vi "Global INIT.vi"() -> ()   [LabVIEW 2023]
uses:
  ctrl defs/ctrl arm motor.ctl
  ctrl defs/ctrl swerve motor.ctl
  ctrl defs/ctrl MOTOR SELECT.ctl
  <vilib>/Rock Robotics/WPI/ThirdParty/REV Robotics/REVLib/Typedef/Spark MAX Idle Mode.ctl
  ctrl defs/ctrl Spark MAX current limiting.ctl
  ctrl defs/ctrl motor PIDF coefficients.ctl
  <vilib>/Rock Robotics/WPI/ThirdParty/REV Robotics/REVLib/Typedef/Spark MAX Smart Motion Parameters.ctl
  ctrl defs/ctrl limit polarity.ctl
  <vilib>/Rock Robotics/WPI/ThirdParty/REV Robotics/REVLib/Typedef/Spark MAX Limit Switch Polarity.ctl
  ctrl defs/ctrl Talon FX config.ctl
  <vilib>/Rock Robotics/WPI/ThirdParty/Phoenix-LabVIEW/Motor Controller/Controls/CTRE_Phoenix_MotorControl_TalonFXInvertType.ctl
  <vilib>/Rock Robotics/WPI/ThirdParty/Phoenix-LabVIEW/Motor Controller/Controls/CTRE_Phoenix_MotorControl_NeutralMode.ctl
  ctrl defs/ctrl CANcoder.ctl
  ctrl defs/ctrl robot CG.ctl
  ctrl defs/ctrl XY coord.ctl
  ctrl defs/ctrl robot swerve dims.ctl
  ctrl defs/ctrl compressor begin.ctl
  ctrl defs/ctrl compressor config.ctl
  <vilib>/Rock Robotics/WPI/Compressor/WPI_CompressorFeedbackMode.ctl
  ctrl defs/ctrl solenoid.ctl
  <vilib>/Rock Robotics/WPI/Solenoid/WPI_SolenoidChannel.ctl
  <vilib>/Rock Robotics/WPI/Solenoid/WPI_SolenoidValue.ctl
  ctrl defs/ctrl DIO.ctl
  <vilib>/Rock Robotics/SystemInterfaces/DIO/FPGA_DIOChannel.ctl
  ctrl defs/ctrl LED init.ctl
  <vilib>/Rock Robotics/SystemInterfaces/DIO/FPGA_DIOPWMChannel.ctl
  ctrl defs/ctrl number of LEDs.ctl
  ctrl defs/ctrl LED PATTERNS.ctl
  ctrl defs/ctrl DEFINE GEAR.ctl
  ctrl defs/ctrl intake speeds.ctl
  ctrl defs/ctrl shooter speeds.ctl
  ctrl defs/ctrl LIMELIGHT initialize.ctl
  ctrl defs/ctrl ctre pigeon2 config.ctl
  <vilib>/Rock Robotics/WPI/ThirdParty/Phoenix-LabVIEW/Pigeon2/controls/CTRE_Phoenix_Pigeon2_Configurables.ctl
panel:
  in  "Tab Control":T1(tab)
  in  "swerve DRIVE motors":T2[](array[typedef])=[{"refnum name"="front right", "CAN ID"=3, "Installed?"=TRUE, "description"="DRIVE - front right ", "MOTOR SELECT"=6000, "CAN Bus"="SWERVE", "Invert Type"=enum."Counter-Clockwise", "Neutral Mode"=enum."Override to Coast", "gear ratio"=6.75, "MOTOR PIDF coefficients"={"PIDF"={"P Gain"=0.001, "I Gain"=0.0, "D Gain"=0.0, "F Gain"=0.0012, "I Zone"=0.0, "Min Output"=-1.0, "Max Output"=1.0}, "Smart Motion"={"Max Velocity"=1900.0, "Max Acceleration"=750.0, "Minimum Velocity Output"=0.1, "Allowed Closed Loop Error"=0.02}}, "Throttle"={"Ramp Open (s)"=0.0, "Ramp Closed (s)"=0.0, "Percent Deadband"=0.0}, "Supply Current Limits"={"Enable?"=FALSE, "Current Limit"=0.0, "Threshold Current"=0.0, "Threshold Time"=0.0}}, {"refnum name"="front left", "CAN ID"=6, "Installed?"=TRUE, "description"="DRIVE - front left", "MOTOR SELECT"=6000, "CAN Bus"="SWERVE", "Invert Type"=enum."Counter-Clockwise", "Neutral Mode"=enum."Override to Coast", "gear ratio"=6.75, "MOTOR PIDF coefficients"={"PIDF"={"P Gain"=0.001, "I Gain"=0.0, "D Gain"=0.0, "F Gain"=0.0012, "I Zone"=0.0, "Min Output"=-1.0, "Max Output"=1.0}, "Smart Motion"={"Max Velocity"=1900.0, "Max Acceleration"=750.0, "Minimum Velocity Output"=0.1, "Allowed Closed Loop Error"=0.02}}, "Throttle"={"Ramp Open (s)"=0.0, "Ramp Closed (s)"=0.0, "Percent Deadband"=0.0}, "Supply Current Limits"={"Enable?"=FALSE, "Current Limit"=0.0, "Threshold Current"=0.0, "Threshold Time"=0.0}}, {"refnum name"="rear left", "CAN ID"=9, "Installed?"=TRUE, "description"="DRIVE - rear left", "MOTOR SELECT"=6000, "CAN Bus"="SWERVE", "Invert Type"=enum."Counter-Clockwise", "Neutral Mode"=enum."Override to Coast", "gear ratio"=6.75, "MOTOR PIDF coefficients"={"PIDF"={"P Gain"=0.001, "I Gain"=0.0, "D Gain"=0.0, "F Gain"=0.0012, "I Zone"=0.0, "Min Output"=-1.0, "Max Output"=1.0}, "Smart Motion"={"Max Velocity"=1900.0, "Max Acceleration"=750.0, "Minimum Velocity Output"=0.1, "Allowed Closed Loop Error"=0.02}}, "Throttle"={"Ramp Open (s)"=0.0, "Ramp Closed (s)"=0.0, "Percent Deadband"=0.0}, "Supply Current Limits"={"Enable?"=FALSE, "Current Limit"=0.0, "Threshold Current"=0.0, "Threshold Time"=0.0}}, {"refnum name"="rear right", "CAN ID"=12, "Installed?"=TRUE, "description"="DRIVE - rear right", "MOTOR SELECT"=6000, "CAN Bus"="SWERVE", "Invert Type"=enum."Counter-Clockwise", "Neutral Mode"=enum."Override to Coast", "gear ratio"=6.75, "MOTOR PIDF coefficients"={"PIDF"={"P Gain"=0.001, "I Gain"=0.0, "D Gain"=0.0, "F Gain"=0.0012, "I Zone"=0.0, "Min Output"=-1.0, "Max Output"=1.0}, "Smart Motion"={"Max Velocity"=1900.0, "Max Acceleration"=750.0, "Minimum Velocity Output"=0.1, "Allowed Closed Loop Error"=0.02}}, "Throttle"={"Ramp Open (s)"=0.0, "Ramp Closed (s)"=0.0, "Percent Deadband"=0.0}, "Supply Current Limits"={"Enable?"=FALSE, "Current Limit"=0.0, "Threshold Current"=0.0, "Threshold Time"=0.0}}] {"gear ratio" format="%_5f"; "MOTOR SELECT" items=["REV NEO"=5676, "REV NEO 550"=11000, "VEX Falcon"=6380, "WC Kraken"=6000]}
  in  "DRIVE\nwheel diam (in)":dbl=4.0 format="%_4f"
  in  "swerve CANcoders":T8[](array[typedef])=[{"description"="ENC - front right", "Installed?"=TRUE, "CAN ID"=2, "CAN Bus"="SWERVE", "refnum name"="FR ENC", "Sensor Direction"=FALSE, "Magnet Offset (Degrees)"=-264.1113, "gear ratio"=1.0}, {"description"="ENC - front left", "Installed?"=TRUE, "CAN ID"=5, "CAN Bus"="SWERVE", "refnum name"="FL ENC", "Sensor Direction"=FALSE, "Magnet Offset (Degrees)"=-277.20703, "gear ratio"=1.0}, {"description"="ENC - rear left", "Installed?"=TRUE, "CAN ID"=8, "CAN Bus"="SWERVE", "refnum name"="RL ENC", "Sensor Direction"=FALSE, "Magnet Offset (Degrees)"=-124.014, "gear ratio"=1.0}, {"description"="ENC - rear right", "Installed?"=TRUE, "CAN ID"=11, "CAN Bus"="SWERVE", "refnum name"="RR ENC", "Sensor Direction"=FALSE, "Magnet Offset (Degrees)"=-162.158, "gear ratio"=1.0}] {"gear ratio" format="%_5f"}
  in  "swerve STEER motors":T9[](array[typedef])=[{"description"="STEER - front right", "MOTOR SELECT"=5676, "Installed?"=TRUE, "CAN ID"=4, "refnum name"="FR STEER", "Invert"=TRUE, "Idle Mode"=enum."Brake", "Current limiting"={"Linearized"=FALSE, "Free Speed (A)"=20.0, "Primay (A)"=40.0, "Limit RPM (0)"=0}, "MOTOR PIDF coefficients"={"PIDF"={"P Gain"=0.005, "I Gain"=0.0, "D Gain"=0.0, "F Gain"=0.0036, "I Zone"=0.0, "Min Output"=-1.0, "Max Output"=1.0}, "Smart Motion"={"Max Velocity"=1500.0, "Max Acceleration"=750.0, "Minimum Velocity Output"=0.1, "Allowed Closed Loop Error"=0.02}}, "gear ratio"=21.42857}, {"description"="STEER - front left", "MOTOR SELECT"=5676, "Installed?"=TRUE, "CAN ID"=7, "refnum name"="FL STEER", "Invert"=TRUE, "Idle Mode"=enum."Brake", "Current limiting"={"Linearized"=FALSE, "Free Speed (A)"=20.0, "Primay (A)"=40.0, "Limit RPM (0)"=0}, "MOTOR PIDF coefficients"={"PIDF"={"P Gain"=0.005, "I Gain"=0.0, "D Gain"=0.0, "F Gain"=0.0036, "I Zone"=0.0, "Min Output"=-1.0, "Max Output"=1.0}, "Smart Motion"={"Max Velocity"=1500.0, "Max Acceleration"=750.0, "Minimum Velocity Output"=0.1, "Allowed Closed Loop Error"=0.02}}, "gear ratio"=21.429}, {"description"="STEER - rear left", "MOTOR SELECT"=5676, "Installed?"=TRUE, "CAN ID"=10, "refnum name"="RL STEER", "Invert"=TRUE, "Idle Mode"=enum."Brake", "Current limiting"={"Linearized"=FALSE, "Free Speed (A)"=20.0, "Primay (A)"=40.0, "Limit RPM (0)"=0}, "MOTOR PIDF coefficients"={"PIDF"={"P Gain"=0.005, "I Gain"=0.0, "D Gain"=0.0, "F Gain"=0.0036, "I Zone"=0.0, "Min Output"=-1.0, "Max Output"=1.0}, "Smart Motion"={"Max Velocity"=1500.0, "Max Acceleration"=750.0, "Minimum Velocity Output"=0.1, "Allowed Closed Loop Error"=0.02}}, "gear ratio"=21.42857}, {"description"="STEER - rear right", "MOTOR SELECT"=5676, "Installed?"=TRUE, "CAN ID"=13, "refnum name"="RR STEER", "Invert"=TRUE, "Idle Mode"=enum."Brake", "Current limiting"={"Linearized"=FALSE, "Free Speed (A)"=20.0, "Primay (A)"=40.0, "Limit RPM (0)"=0}, "MOTOR PIDF coefficients"={"PIDF"={"P Gain"=0.005, "I Gain"=0.0, "D Gain"=0.0, "F Gain"=0.0036, "I Zone"=0.0, "Min Output"=-1.0, "Max Output"=1.0}, "Smart Motion"={"Max Velocity"=1500.0, "Max Acceleration"=750.0, "Minimum Velocity Output"=0.1, "Allowed Closed Loop Error"=0.02}}, "gear ratio"=21.42857}] {"gear ratio" format="%_5f"; "MOTOR SELECT" items=["REV NEO"=5676, "REV NEO 550"=11000, "VEX Falcon"=6380, "WC Kraken"=6000]}
  in  "PIGEON":T12={"Installed?"=TRUE, "Configurables"={"Mount Pose Yaw"=0.0, "Mount Pose Pitch"=0.0, "Mount Pose Roll"=0.0, "Disable Temperature Compensation"=FALSE, "Disable No-Motion Calibration"=FALSE, "Enable Compass"=TRUE}, "CAN ID"=1, "refnum name"="PIGEON2", "CAN bus"="SWERVE"}
  in  "LIMELIGHT":T14={"Installed?"=TRUE, "pose"={"X"=0.0, "Y"=-3.0, "Z"=23.0, "angle to horizon"=-34.5, "tx angle offset"=0.0}}
  in  "LED init":T15={"PWM Channel"=enum."PWM 1", "refnum name"="LED", "#LEDS"=120, "initial output"=0.51, "stack name"="LED/value", "Installed?"=TRUE, "pattern"=0} {"pattern" items=["<<Select a pattern>>", "Rainbow, Rainbow palette", "Rainbow, Party palette", "Rainbow, Ocean palette", "Rainbow, Lava palette", "Rainbow, Forest palette", "Rainbow with glitter", "Confetti", "Shot, Red", "Shot, Blue", "Shot, White", "Sinelon, Rainbow palette", "Sinelon, Party palette", "Sinelon, Ocean palette", "Sinelon, Lava palette", "Sinelon, Forest palette", "BPM, Rainbow palette", "BPM, Party palette", "BPM, Ocean palette", "BPM, Lava palette", "BPM, Forest palette", "Fire, Medium", "Fire, Large", "Twinkles, Rainbow palette", "Twinkles, Party palette", "Twinkles, Ocean palette", "Twinkles, Lava palette", "Twinkles, Forest palette", "Color Waves, Rainbow palette", "Color Waves, Party palette", "Color Waves, Ocean palette", "Color Waves, Lava palette", "Color Waves, Forest palette", "Larson Scanner, Red", "Larson Scanner, Gray", "Light Chase, Red", "Light Chase, Blue", "Light Chase, Gray", "Heartbeat, Red", "Heartbeat, Blue", "Heartbeat, White", "Heartbeat, Gray", "Breath, Red", "Breath, Blue", "Breath, Gray", "Strobe, Red", "Strobe, Blue", "Strobe, Gold", "Strobe, White", "Color 1: End to End Blend to Black", "Color 1: Larson Scanner", "Color 1: Light Chase", "Color 1: Heartbeat Slow", "Color 1: Heartbeat Medium", "Color 1: Heartbeat Fast", "Color 1: Breath Slow", "Color 1: Breath Fast", "Color 1: Shot", "Color 1: Strobe", "Color 2: End to End Blend to Black", "Color 2: Larson Scanner", "Color 2: Light Chase", "Color 2: Heartbeat Slow", "Color 2: Heartbeat Medium", "Color 2: Heartbeat Fast", "Color 2: Breath Slow", "Color 2: Breath Fast", "Color 2: Shot", "Color 2: Strobe", "Color 1/2: Sparkle, 1 on 2", "Color 1/2: Sparkle 2 on 1", "Color 1/2: Gradient", "Color 1/2: BPM", "Color 1/2: End to End Blend 1 to 2", "Color 1/2: End to End Blend 2 to 1", "Color 1/2: setup pattern", "Color 1/2: Twinkles", "Color 1/2: Color Waves", "Color 1/2: Sinelon", "Solid Hot Pink", "Solid Dark Red", "Solid Red", "Solid Red Orange", "Solid Orange", "Solid Gold", "Solid Yellow", "Solid Lawn Green", "Solid Lime", "Solid Dark Green", "Solid Green", "Solid Blue Green", "Solid Aqua", "Solid Sky Blue", "Solid Dark Blue", "Solid Blue", "Solid Blue Violet", "Solid Violet", "Solid White", "Solid Gray", "Solid Dark Gray", "Solid Black"]}
  in  "DIO":T19[](array[typedef])=[{"description"="NOTE color sensor", "Installed?"=TRUE, "DIOChannel"=enum."DIO 0", "refnum name"="ref COLOR"}]
  in  "IMU OFFSET (deg)":dbl=90.0 format="%_4f"
  in  "ROBOT frame dims":T21={"width"=30.0, "depth"=30.0}
  in  "swerve position coeff":T22(array[cluster])=[{"description"="front right", "wrt geom CTR"={"delX"=1, "delY"=1}}, {"description"="front left", "wrt geom CTR"={"delX"=-1, "delY"=1}}, {"description"="rear left", "wrt geom CTR"={"delX"=-1, "delY"=-1}}, {"description"="rear right", "wrt geom CTR"={"delX"=1, "delY"=-1}}]
  in  "ROBOT swerve dims":T21={"width"=24.75, "depth"=24.75}
  in  "ROBOT CG":T23={"mass (lbm)"=138.0, "CG"={"X"=-0.2832231884057969, "Y"=-0.6018492753623189}, "Zcg"=24.0} {"CG"."Y" format="%.4g"; "CG"."X" format="%.4g"}
  in  "SOLENOIDS":T25[](array[typedef])=[{"description"="arm lock - BOTH", "Installed?"=TRUE, "refnum name"="LOCK - LEFT", "coils"=enum."Double", "forward channel"=enum."Solenoid 2", "reverse channel"=enum."Solenoid 3", "initial value"=enum."Reverse"}, {"description"="FLAP", "Installed?"=TRUE, "refnum name"="FLAP", "coils"=enum."Double", "forward channel"=enum."Solenoid 1", "reverse channel"=enum."Solenoid 0", "initial value"=enum."Reverse"}]
  in  "COMPRESSOR":T28={"description"="compressor", "Installed?"=TRUE, "refnum name"="COMP", "Feedback Configuration"={"Feedback Sensor"=enum."Digital Only", "Max Pressure (PSI)"=0.0, "Min Pressure (PSI)"=0.0}}
  in  "INTAKE speeds":T31={"forward"=1.0, "reverse"=-1.0} {"reverse" min=-1.0 max=-0.02 format="%.3f"; "forward" min=0.02 max=1.0 format="%.3f"}
  in  "INTAKE motor":T9={"description"="INTAKE", "MOTOR SELECT"=5676, "Installed?"=TRUE, "CAN ID"=11, "refnum name"="ref INTAKE", "Invert"=FALSE, "Idle Mode"=enum."Brake", "Current limiting"={"Linearized"=FALSE, "Free Speed (A)"=20.0, "Primay (A)"=40.0, "Limit RPM (0)"=0}, "MOTOR PIDF coefficients"={"PIDF"={"P Gain"=0.001, "I Gain"=0.0, "D Gain"=0.0, "F Gain"=0.0012, "I Zone"=0.0, "Min Output"=-1.0, "Max Output"=1.0}, "Smart Motion"={"Max Velocity"=1900.0, "Max Acceleration"=750.0, "Minimum Velocity Output"=0.1, "Allowed Closed Loop Error"=0.02}}, "gear ratio"=4.0} {"gear ratio" format="%_5f"; "MOTOR SELECT" items=["REV NEO"=5676, "REV NEO 550"=11000, "VEX Falcon"=6380, "WC Kraken"=6000]}
  in  "INTAKE GEAR TRAIN":T32[](array[typedef])=[{"DP"=20.0, "TEETH"=48, "DIAM (in)"=2.4, "rev"=FALSE, "ratio"=1.0}, {"DP"=20.0, "TEETH"=48, "DIAM (in)"=2.4, "rev"=TRUE, "ratio"=-1.0}, {"DP"=20.0, "TEETH"=20, "DIAM (in)"=1.0, "rev"=FALSE, "ratio"=0.4166666666666667}, {"DP"=20.0, "TEETH"=32, "DIAM (in)"=1.6, "rev"=TRUE, "ratio"=-0.6666666666666666}, {"DP"=20.0, "TEETH"=48, "DIAM (in)"=2.4, "rev"=FALSE, "ratio"=1.0}]
  in  "INTAKE ratio TO SMALL WHEEL":dbl=4.0
  in  "INTAKE ratio TO LARGE WHEEL":dbl=4.0
  in  "INTAKE wheel diam (in) - SM":dbl=2.25
  in  "INTAKE wheel diam (in) - LG":dbl=4.0
  out "K INTAKE":dbl=1.0 format="%#_13g"
  out "K LOADER":dbl=0.7272727272727272 format="%#_13g"
  in  "SHOOTER speeds":T33={"SPEAKER"=1.0, "AMP"=0.08} {"AMP" min=0.02 max=1.0 format="%.3f"; "SPEAKER" min=0.02 max=1.0 format="%.3f"}
  in  "DISABLE SHOOTER MECH":bool
  in  "SHOOTING motors":T9[](array[typedef])=[{"description"="SHOOTER CW MOTOR", "MOTOR SELECT"=5676, "Installed?"=TRUE, "CAN ID"=13, "refnum name"="ref SHOOTER", "Invert"=TRUE, "Idle Mode"=enum."Brake", "Current limiting"={"Linearized"=FALSE, "Free Speed (A)"=20.0, "Primay (A)"=40.0, "Limit RPM (0)"=0}, "MOTOR PIDF coefficients"={"PIDF"={"P Gain"=0.001, "I Gain"=0.0, "D Gain"=0.0, "F Gain"=0.0012, "I Zone"=0.0, "Min Output"=-1.0, "Max Output"=1.0}, "Smart Motion"={"Max Velocity"=1900.0, "Max Acceleration"=750.0, "Minimum Velocity Output"=0.1, "Allowed Closed Loop Error"=0.02}}, "gear ratio"=1.0}, {"description"="SHOOTER CCW follow", "MOTOR SELECT"=5676, "Installed?"=TRUE, "CAN ID"=14, "refnum name"="ref SHOOTER follow", "Invert"=TRUE, "Idle Mode"=enum."Brake", "Current limiting"={"Linearized"=FALSE, "Free Speed (A)"=20.0, "Primay (A)"=40.0, "Limit RPM (0)"=0}, "MOTOR PIDF coefficients"={"PIDF"={"P Gain"=0.001, "I Gain"=0.0, "D Gain"=0.0, "F Gain"=0.0012, "I Zone"=0.0, "Min Output"=-1.0, "Max Output"=1.0}, "Smart Motion"={"Max Velocity"=1900.0, "Max Acceleration"=750.0, "Minimum Velocity Output"=0.1, "Allowed Closed Loop Error"=0.02}}, "gear ratio"=1.0}] {"gear ratio" format="%_5f"; "MOTOR SELECT" items=["REV NEO"=5676, "REV NEO 550"=11000, "VEX Falcon"=6380, "WC Kraken"=6000]}
  in  "SHOOTER wheel diam (in)":dbl=4.0
  in  "ARM speeds":T31={"forward"=0.75, "reverse"=-0.5} {"reverse" min=-1.0 max=-0.02 format="%.3f"; "forward" min=0.02 max=1.0 format="%.3f"}
  in  "ARM motors":T34[](array[typedef])=[{" motor"={"description"="ARM-LEFT", "MOTOR SELECT"=5676, "Installed?"=TRUE, "CAN ID"=17, "refnum name"="ref ARM L", "Invert"=TRUE, "Idle Mode"=enum."Brake", "Current limiting"={"Linearized"=FALSE, "Free Speed (A)"=20.0, "Primay (A)"=40.0, "Limit RPM (0)"=0}, "MOTOR PIDF coefficients"={"PIDF"={"P Gain"=0.001, "I Gain"=0.0, "D Gain"=0.0, "F Gain"=0.0012, "I Zone"=0.0, "Min Output"=-1.0, "Max Output"=1.0}, "Smart Motion"={"Max Velocity"=1900.0, "Max Acceleration"=750.0, "Minimum Velocity Output"=0.1, "Allowed Closed Loop Error"=0.02}}, "gear ratio"=16.0}, "limit polarities"={"Forward limit"=enum."Normally Closed", "Reverse limit"=enum."Normally Closed"}}, {" motor"={"description"="ARM-RIGHT", "MOTOR SELECT"=5676, "Installed?"=TRUE, "CAN ID"=16, "refnum name"="ref ARM R", "Invert"=FALSE, "Idle Mode"=enum."Brake", "Current limiting"={"Linearized"=FALSE, "Free Speed (A)"=20.0, "Primay (A)"=40.0, "Limit RPM (0)"=0}, "MOTOR PIDF coefficients"={"PIDF"={"P Gain"=0.001, "I Gain"=0.0, "D Gain"=0.0, "F Gain"=0.0012, "I Zone"=0.0, "Min Output"=-1.0, "Max Output"=1.0}, "Smart Motion"={"Max Velocity"=1900.0, "Max Acceleration"=750.0, "Minimum Velocity Output"=0.1, "Allowed Closed Loop Error"=0.02}}, "gear ratio"=16.0}, "limit polarities"={"Forward limit"=enum."Normally Closed", "Reverse limit"=enum."Normally Closed"}}] {"motor"."gear ratio" format="%_5f"; "motor"."MOTOR SELECT" items=["REV NEO"=5676, "REV NEO 550"=11000, "VEX Falcon"=6380, "WC Kraken"=6000]}
  in  "LOADER max/min":T31={"forward"=1.0, "reverse"=-1.0} {"reverse" min=-1.0 max=-0.02 format="%.3f"; "forward" min=0.02 max=1.0 format="%.3f"}
  in  "LOADER speeds":T31={"forward"=0.85, "reverse"=-1.0} {"reverse" min=-1.0 max=-0.02 format="%.3f"; "forward" min=0.02 max=1.0 format="%.3f"}
  in  "LOADER wheel diam (in)":dbl=2.75
  in  "LOADING motors":T9[](array[typedef])=[{"description"="LOADING CW MOTOR", "MOTOR SELECT"=11000, "Installed?"=TRUE, "CAN ID"=12, "refnum name"="ref LOADER", "Invert"=FALSE, "Idle Mode"=enum."Brake", "Current limiting"={"Linearized"=FALSE, "Free Speed (A)"=20.0, "Primay (A)"=40.0, "Limit RPM (0)"=0}, "MOTOR PIDF coefficients"={"PIDF"={"P Gain"=0.001, "I Gain"=0.0, "D Gain"=0.0, "F Gain"=0.0012, "I Zone"=0.0, "Min Output"=-1.0, "Max Output"=1.0}, "Smart Motion"={"Max Velocity"=1900.0, "Max Acceleration"=750.0, "Minimum Velocity Output"=0.1, "Allowed Closed Loop Error"=0.02}}, "gear ratio"=4.0}, {"description"="LOADING CCW follow", "MOTOR SELECT"=11000, "Installed?"=TRUE, "CAN ID"=15, "refnum name"="ref LOADERS follow", "Invert"=TRUE, "Idle Mode"=enum."Brake", "Current limiting"={"Linearized"=FALSE, "Free Speed (A)"=20.0, "Primay (A)"=40.0, "Limit RPM (0)"=0}, "MOTOR PIDF coefficients"={"PIDF"={"P Gain"=0.001, "I Gain"=0.0, "D Gain"=0.0, "F Gain"=0.0012, "I Zone"=0.0, "Min Output"=-1.0, "Max Output"=1.0}, "Smart Motion"={"Max Velocity"=1900.0, "Max Acceleration"=750.0, "Minimum Velocity Output"=0.1, "Allowed Closed Loop Error"=0.02}}, "gear ratio"=4.0}] {"gear ratio" format="%_5f"; "MOTOR SELECT" items=["REV NEO"=5676, "REV NEO 550"=11000, "VEX Falcon"=6380, "WC Kraken"=6000]}
  # "Yaw Angle needed to reach the current orientation in degrees"
  # "Configures the mounting pose of the Pigeon2\nThis is the yaw-pitch-roll teh Pigeon2 underwent to get to its current orientation,\n referenced from the robot's point of view\nThis is only necessary if the Pigeon2 is mounted at an exotic angle near the gimbal lock point or not forward.\nIf the pigeon is relatively flat and pointed forward, this is not needed"
  # "Pitch Angle needed to reach the current orientation in degrees"
  # "Roll Angle needed to reach the current orientation in degrees"
  # "Disables the temperature compensation\nfrom the Pigeon2. It is recommended that\nthis remains false"
  # "Disables the no-motion calibration from the\nPigeon2. It is recommended that this \nremains false"
  # "Enables the compass for Pigeon2\nThis is not recommended for any indoor robotics"
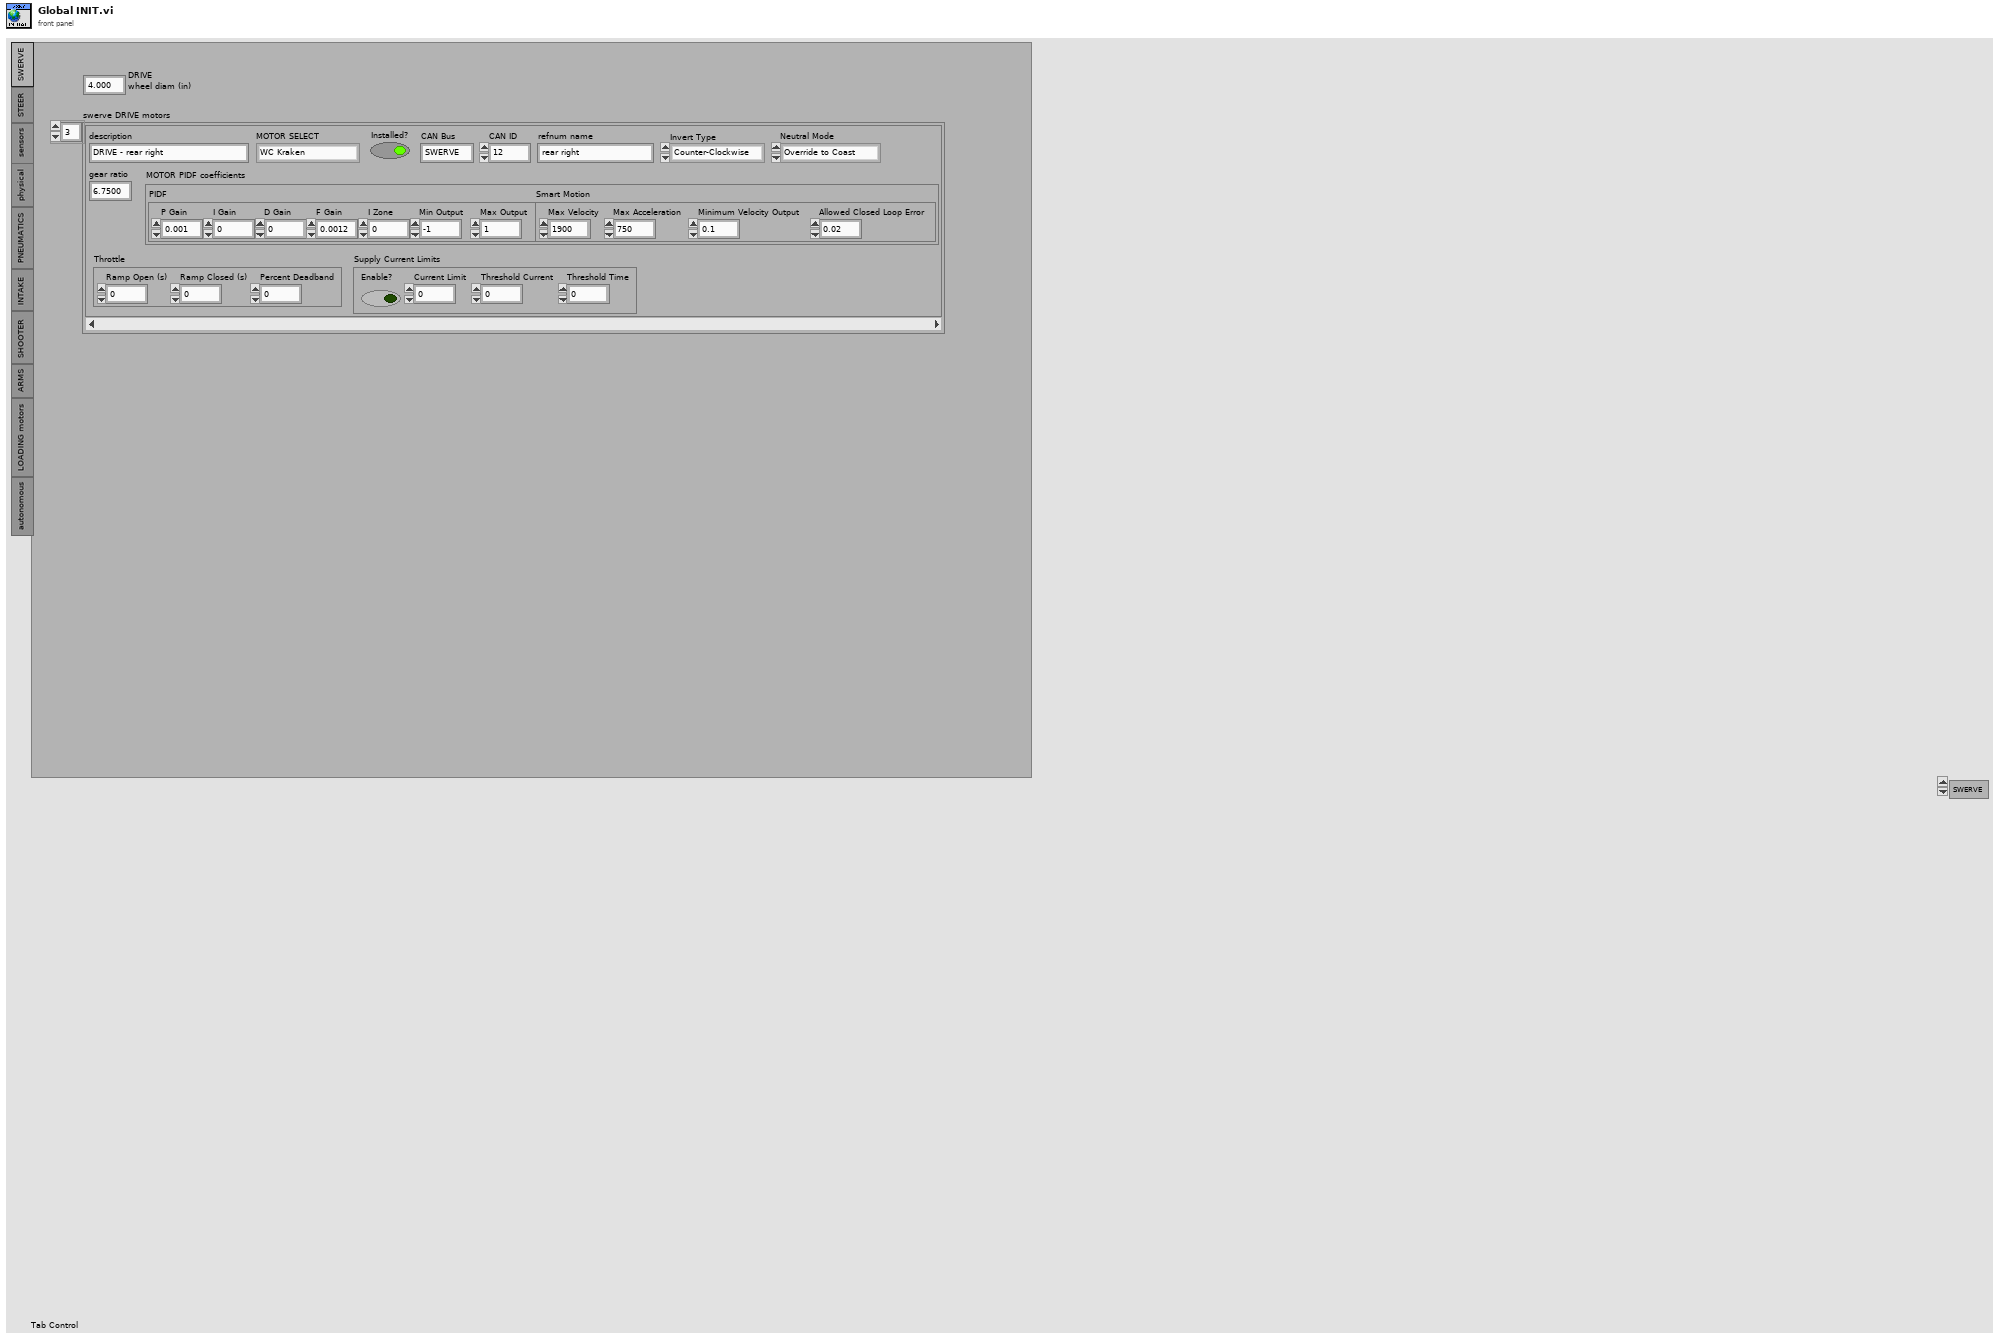
[diagram p1: front panel]
types:
  T1 = enum32{"SWERVE", "STEER", "sensors", "physical", "PNEUMATICS", "INTAKE ", "SHOOTER ", "ARMS", "LOADING motors", "autonomous"}
  T2 = typedef "ctrl Talon FX config.ctl" = cluster{"refnum name":string, "CAN ID":u8, "Installed?":bool, "description":string, "MOTOR SELECT":T3, "CAN Bus":string, "Invert Type":T4, "Neutral Mode":T5, "gear ratio":dbl, "MOTOR PIDF coefficients":T6, "Throttle":cluster{"Ramp Open (s)":dbl, "Ramp Closed (s)":dbl, "Percent Deadband":dbl}, "Supply Current Limits":cluster{"Enable?":bool, "Current Limit":dbl, "Threshold Current":dbl, "Threshold Time":dbl}}
  T3 = typedef "ctrl MOTOR SELECT.ctl" = i16
  T4 = typedef "CTRE_Phoenix_MotorControl_TalonFXInvertType.ctl" = enum16{"Counter-Clockwise", "Clockwise"}
  T5 = typedef "CTRE_Phoenix_MotorControl_NeutralMode.ctl" = enum8{"EEPROMSetting", "Override to Coast", "Override to Brake"}
  T6 = typedef "ctrl motor PIDF coefficients.ctl" = cluster{"PIDF":cluster{"P Gain":dbl, "I Gain":dbl, "D Gain":dbl, "F Gain":dbl, "I Zone":dbl, "Min Output":dbl, "Max Output":dbl}, "Smart Motion":T7}
  T7 = typedef "Spark MAX Smart Motion Parameters.ctl" = cluster{"Max Velocity":dbl, "Max Acceleration":dbl, "Minimum Velocity Output":dbl, "Allowed Closed Loop Error":dbl}
  T8 = typedef "ctrl CANcoder.ctl" = cluster{"description":string, "Installed?":bool, "CAN ID":u8, "CAN Bus":string, "refnum name":string, "Sensor Direction":bool, "Magnet Offset (Degrees)":dbl, "gear ratio":dbl}
  T9 = typedef "ctrl swerve motor.ctl" = cluster{"description":string, "MOTOR SELECT":T3, "Installed?":bool, "CAN ID":u8, "refnum name":string, "Invert":bool, "Idle Mode":T10, "Current limiting":T11, "MOTOR PIDF coefficients":T6, "gear ratio":dbl}
  T10 = typedef "Spark MAX Idle Mode.ctl" = enum16{"Coast", "Brake"}
  T11 = typedef "ctrl Spark MAX current limiting.ctl" = cluster{"Linearized":bool, "Free Speed (A)":dbl, "Primay (A)":dbl, "Limit RPM (0)":u32}
  T12 = typedef "ctrl ctre pigeon2 config.ctl" = cluster{"Installed?":bool, "Configurables":T13, "CAN ID":u8, "refnum name":string, "CAN bus":string}
  T13 = typedef "CTRE_Phoenix_Pigeon2_Configurables.ctl" = cluster{"Mount Pose Yaw":dbl, "Mount Pose Pitch":dbl, "Mount Pose Roll":dbl, "Disable Temperature Compensation":bool, "Disable No-Motion Calibration":bool, "Enable Compass":bool}
  T14 = typedef "ctrl LIMELIGHT initialize.ctl" = cluster{"Installed?":bool, "pose":cluster{"X":dbl, "Y":dbl, "Z":dbl, "angle to horizon":dbl, "tx angle offset":dbl}}
  T15 = typedef "ctrl LED init.ctl" = cluster{"PWM Channel":T16, "refnum name":string, "#LEDS":T17, "initial output":dbl, "stack name":string, "Installed?":bool, "pattern":T18}
  T16 = typedef "FPGA_DIOPWMChannel.ctl" = enum8{"PWM 0", "PWM 1", "PWM 2", "PWM 3", "PWM 4", "PWM 5", "PWM 6", "PWM 7", "PWM 8", "PWM 9", "PWM MXP 0", "PWM MXP 1", "PWM MXP 2", "PWM MXP 3", "PWM MXP 4", "PWM MXP 5", "PWM MXP 6", "PWM MXP 7", "PWM MXP 8", "PWM MXP 9", "Invalid"}
  T17 = typedef "ctrl number of LEDs.ctl" = u16
  T18 = typedef "ctrl LED PATTERNS.ctl" = u16
  T19 = typedef "ctrl DIO.ctl" = cluster{"description":string, "Installed?":bool, "DIOChannel":T20, "refnum name":string}
  T20 = typedef "FPGA_DIOChannel.ctl" = enum8{"DIO 0", "DIO 1", "DIO 2", "DIO 3", "DIO 4", "DIO 5", "DIO 6", "DIO 7", "DIO 8", "DIO 9", "DIO MXP 0", "DIO MXP 1", "DIO MXP 2", "DIO MXP 3", "DIO MXP 4", "DIO MXP 5", "DIO MXP 6", "DIO MXP 7", "DIO MXP 8", "DIO MXP 9", "DIO MXP 10", "DIO MXP 11", "DIO MXP 12", "DIO MXP 13", "DIO MXP 14", "DIO MXP 15", "SPI Port CS1", "SPI Port CS2", "SPI Port CS3", "SPI Port MISO", "SPI Port MOSI", "Invalid"}
  T21 = typedef "ctrl robot swerve dims.ctl" = cluster{"width":dbl, "depth":dbl}
  T22 = cluster{"description":string, "wrt geom CTR":cluster{"delX":i8, "delY":i8}}[]
  T23 = typedef "ctrl robot CG.ctl" = cluster{"mass (lbm)":dbl, "CG":T24, "Zcg":dbl}
  T24 = typedef "ctrl XY coord.ctl" = cluster{"X":dbl, "Y":dbl}
  T25 = typedef "ctrl solenoid.ctl" = cluster{"description":string, "Installed?":bool, "refnum name":string, "coils":enum16{"Single", "Double"}, "forward channel":T26, "reverse channel":T26, "initial value":T27}
  T26 = typedef "WPI_SolenoidChannel.ctl" = enum8{"Solenoid 0", "Solenoid 1", "Solenoid 2", "Solenoid 3", "Solenoid 4", "Solenoid 5", "Solenoid 6", "Solenoid 7", "Solenoid 8", "Solenoid 9", "Solenoid 10", "Solenoid 11", "Solenoid 12", "Solenoid 13", "Solenoid 14", "Solenoid 15", "Invalid"}
  T27 = typedef "WPI_SolenoidValue.ctl" = enum16{"Off", "On", "Forward", "Reverse"}
  T28 = typedef "ctrl compressor begin.ctl" = cluster{"description":string, "Installed?":bool, "refnum name":string, "Feedback Configuration":T29}
  T29 = typedef "ctrl compressor config.ctl" = cluster{"Feedback Sensor":T30, "Max Pressure (PSI)":dbl, "Min Pressure (PSI)":dbl}
  T30 = typedef "WPI_CompressorFeedbackMode.ctl" = enum16{"Analog Only", "Digital Only", "Hybrid"}
  T31 = typedef "ctrl intake speeds.ctl" = cluster{"forward":dbl, "reverse":dbl}
  T32 = typedef "ctrl DEFINE GEAR.ctl" = cluster{"DP":dbl, "TEETH":i16, "DIAM (in)":dbl, "rev":bool, "ratio":dbl}
  T33 = typedef "ctrl shooter speeds.ctl" = cluster{"SPEAKER":dbl, "AMP":dbl}
  T34 = typedef "ctrl arm motor.ctl" = cluster{" motor":T9, "limit polarities":T35}
  T35 = typedef "ctrl limit polarity.ctl" = cluster{"Forward limit":T36, "Reverse limit":T36}
  T36 = typedef "Spark MAX Limit Switch Polarity.ctl" = enum16{"Normally Open", "Normally Closed"}
diagram:
